vi "Update.vi"(10 "Image":variant[][](array[variant]), 11 "Base Graph in":refnum<class "Base Graph.lvclass">) -> (3 "Base Graph out":refnum<class "Base Graph.lvclass">)   [LabVIEW 2023, in "Base Graph.lvclass"]
uses:
  Base Graph.lvclass
  Base Graph.lvclass/Base Graph.ctl
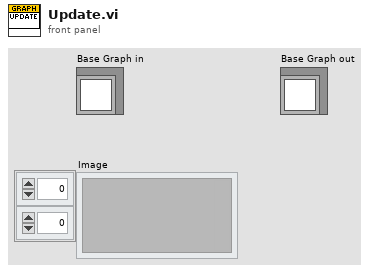
[diagram p1: front panel]
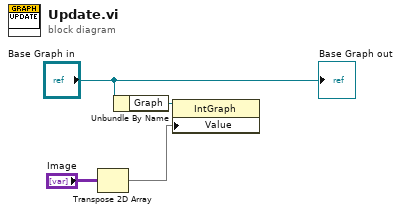
[diagram p0: block diagram]
diagram:
  n1 = Transpose 2D Array(2D array="Image") -> (transposed array=w2:variant[][])
  n2 = Unbundle By Name("Base Graph in") -> ("Graph"=w3:refnum<vi>)
  n3 = property class="IntGraph"(reference=w3, "Value"=w2) -> ()  [unwired: 1 in, 2 out]
  "Base Graph out" <- "Base Graph in"
